vi "calc_jumpTrainWaveform_v0.03.vi"(0 "New input cluster":T1={"Which Position to use for Experiment"=enum."Jumper Safe Position", "Start Position (N)"="", "Jump Position (m)"="", "Duration (s)"=0.0, "Delay (s)"=0.0, "Pulse Width (s)"=0.0, "Valve 1 Position"=0, "Valve 2 Position"=0, "Replicates"=0.0, "Pulse Period (s)"=0.0, "Vholding (mV)"=1.0, "Number of Pulses"=1.0, "valve 1 used now?"=FALSE, "valve 2 used now?"=FALSE, "valve 3 used now? "=FALSE, "Valve 3 Position"=1, "protocol Preview"=[]} {"Valve 3 Position" min=1 max=8; "Number of Pulses" min=1.0 max=8.0; "Vholding (mV)" min=1.0 max=8.0}, 1 "Clear Waveform?":bool, 5 "Old input cluster":T1={"Which Position to use for Experiment"=enum."Jumper Safe Position", "Start Position (N)"="", "Jump Position (m)"="", "Duration (s)"=0.0, "Delay (s)"=0.0, "Pulse Width (s)"=0.0, "Valve 1 Position"=0, "Valve 2 Position"=0, "Replicates"=0.0, "Pulse Period (s)"=0.0, "Vholding (mV)"=1.0, "Number of Pulses"=1.0, "valve 1 used now?"=FALSE, "valve 2 used now?"=FALSE, "valve 3 used now? "=FALSE, "Valve 3 Position"=1, "protocol Preview"=[]} {"Valve 3 Position" min=1 max=8; "Number of Pulses" min=1.0 max=8.0; "Vholding (mV)" min=1.0 max=8.0}, 7 "sample freq":i32=10000, 9 "Jump Filter Freq (Hz)":dbl=30.0, 11 "error in":errorcluster) -> (4 "output cluster":T1={"Which Position to use for Experiment"=enum."Jumper Safe Position", "Start Position (N)"="", "Jump Position (m)"="", "Duration (s)"=0.0, "Delay (s)"=0.0, "Pulse Width (s)"=0.0, "Valve 1 Position"=0, "Valve 2 Position"=0, "Replicates"=0.0, "Pulse Period (s)"=0.0, "Vholding (mV)"=1.0, "Number of Pulses"=1.0, "valve 1 used now?"=FALSE, "valve 2 used now?"=FALSE, "valve 3 used now? "=FALSE, "Valve 3 Position"=1, "protocol Preview"=[]} {"Valve 3 Position" min=1 max=8; "Number of Pulses" min=1.0 max=8.0; "Vholding (mV)" min=1.0 max=8.0}, 15 "error out":errorcluster)   [LabVIEW 2019]
uses:
  <vilib>/Analysis/3filter.llb/Filter Passband Type.ctl
  <vilib>/Analysis/3filter.llb/Bessel Filter (DBL).vi
  <vilib>/measure/NI_MABase.lvlib
  <vilib>/Analysis/NI_AALBase.lvlib
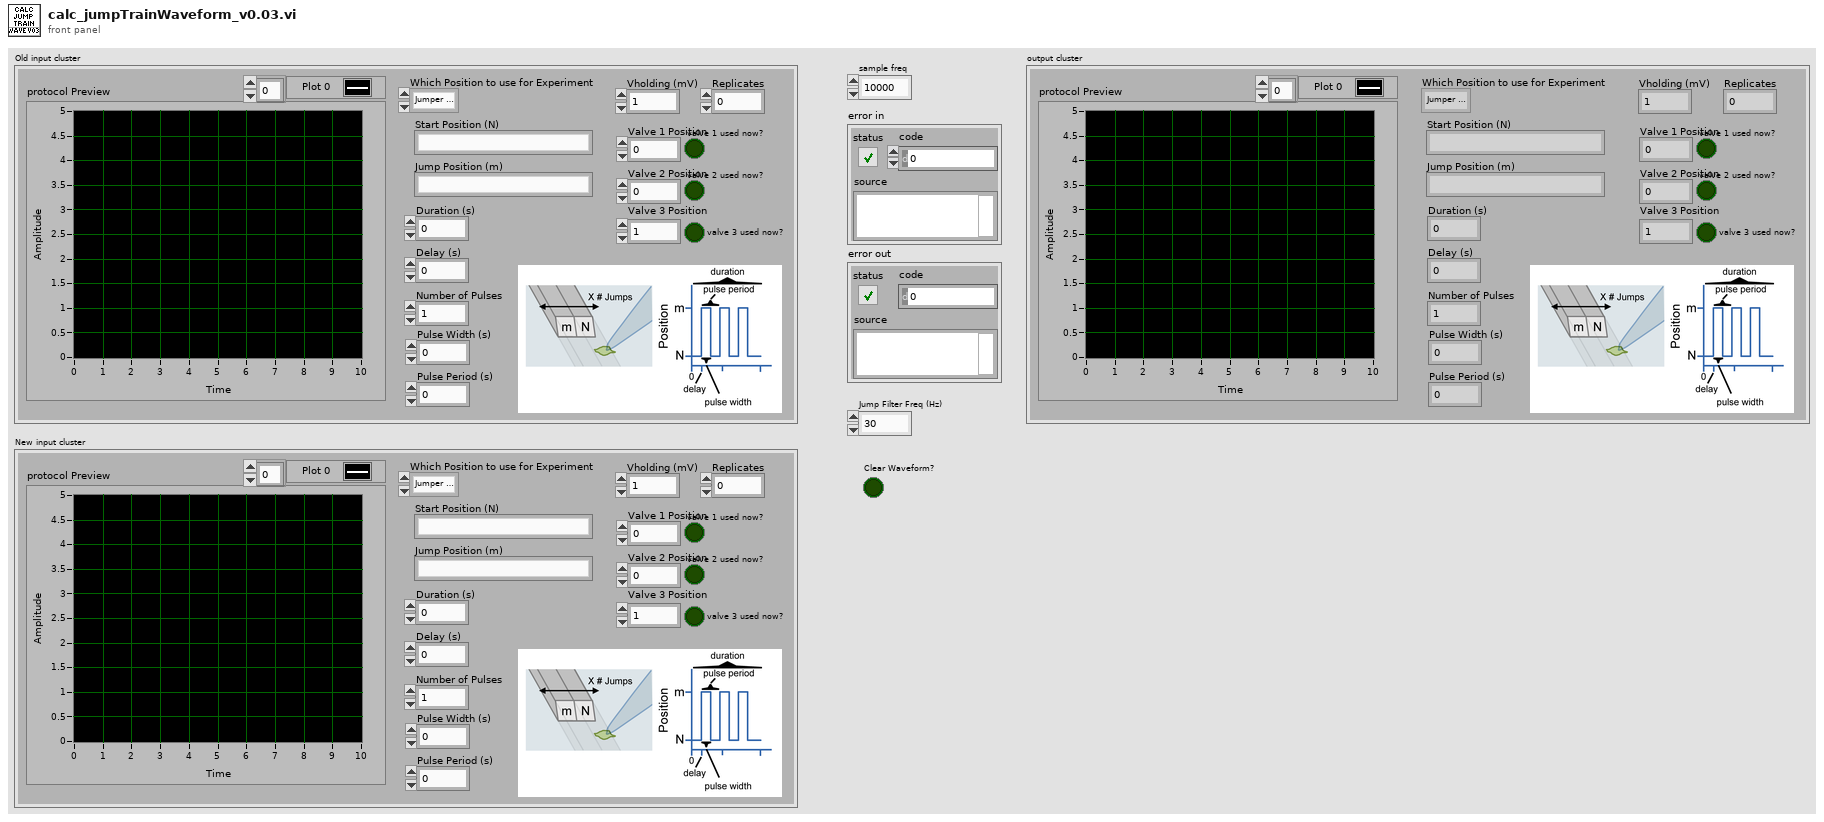
[diagram p1: front panel]
types:
  T1 = cluster{"Which Position to use for Experiment":enum16{"Jumper Safe Position", "Experiment Safe Position", "Jumper Position A", "Jumper Position B", "Jumper Position C", "Jumper Position o-A", "Jumper Position A-o", "Jumper Position A-B", "Jumper Position B-A", "Jumper Position B-C", "Jumper Position C-B", "Jumper Position C-o", "Jumper Position o-C", "Don't Move"}, "Start Position (N)":string, "Jump Position (m)":string, "Duration (s)":dbl, "Delay (s)":dbl, "Pulse Width (s)":dbl, "Valve 1 Position":i16, "Valve 2 Position":i16, "Replicates":dbl, "Pulse Period (s)":dbl, "Vholding (mV)":dbl, "Number of Pulses":dbl, "valve 1 used now?":bool, "valve 2 used now?":bool, "valve 3 used now? ":bool, "Valve 3 Position":i16, "protocol Preview":waveform(dbl)[]}
  T2 = typedef "NI_AALBase.lvlib/Filter Passband Type.ctl" = enum32{"Lowpass", "Highpass", "Bandpass", "Bandstop"}
  T3 = enum16{"Jumper Safe Position", "Experiment Safe Position", "Jumper Position A", "Jumper Position B", "Jumper Position C", "Jumper Position o-A", "Jumper Position A-o", "Jumper Position A-B", "Jumper Position B-A", "Jumper Position B-C", "Jumper Position C-B", "Jumper Position C-o", "Jumper Position o-C", "Don't Move"}
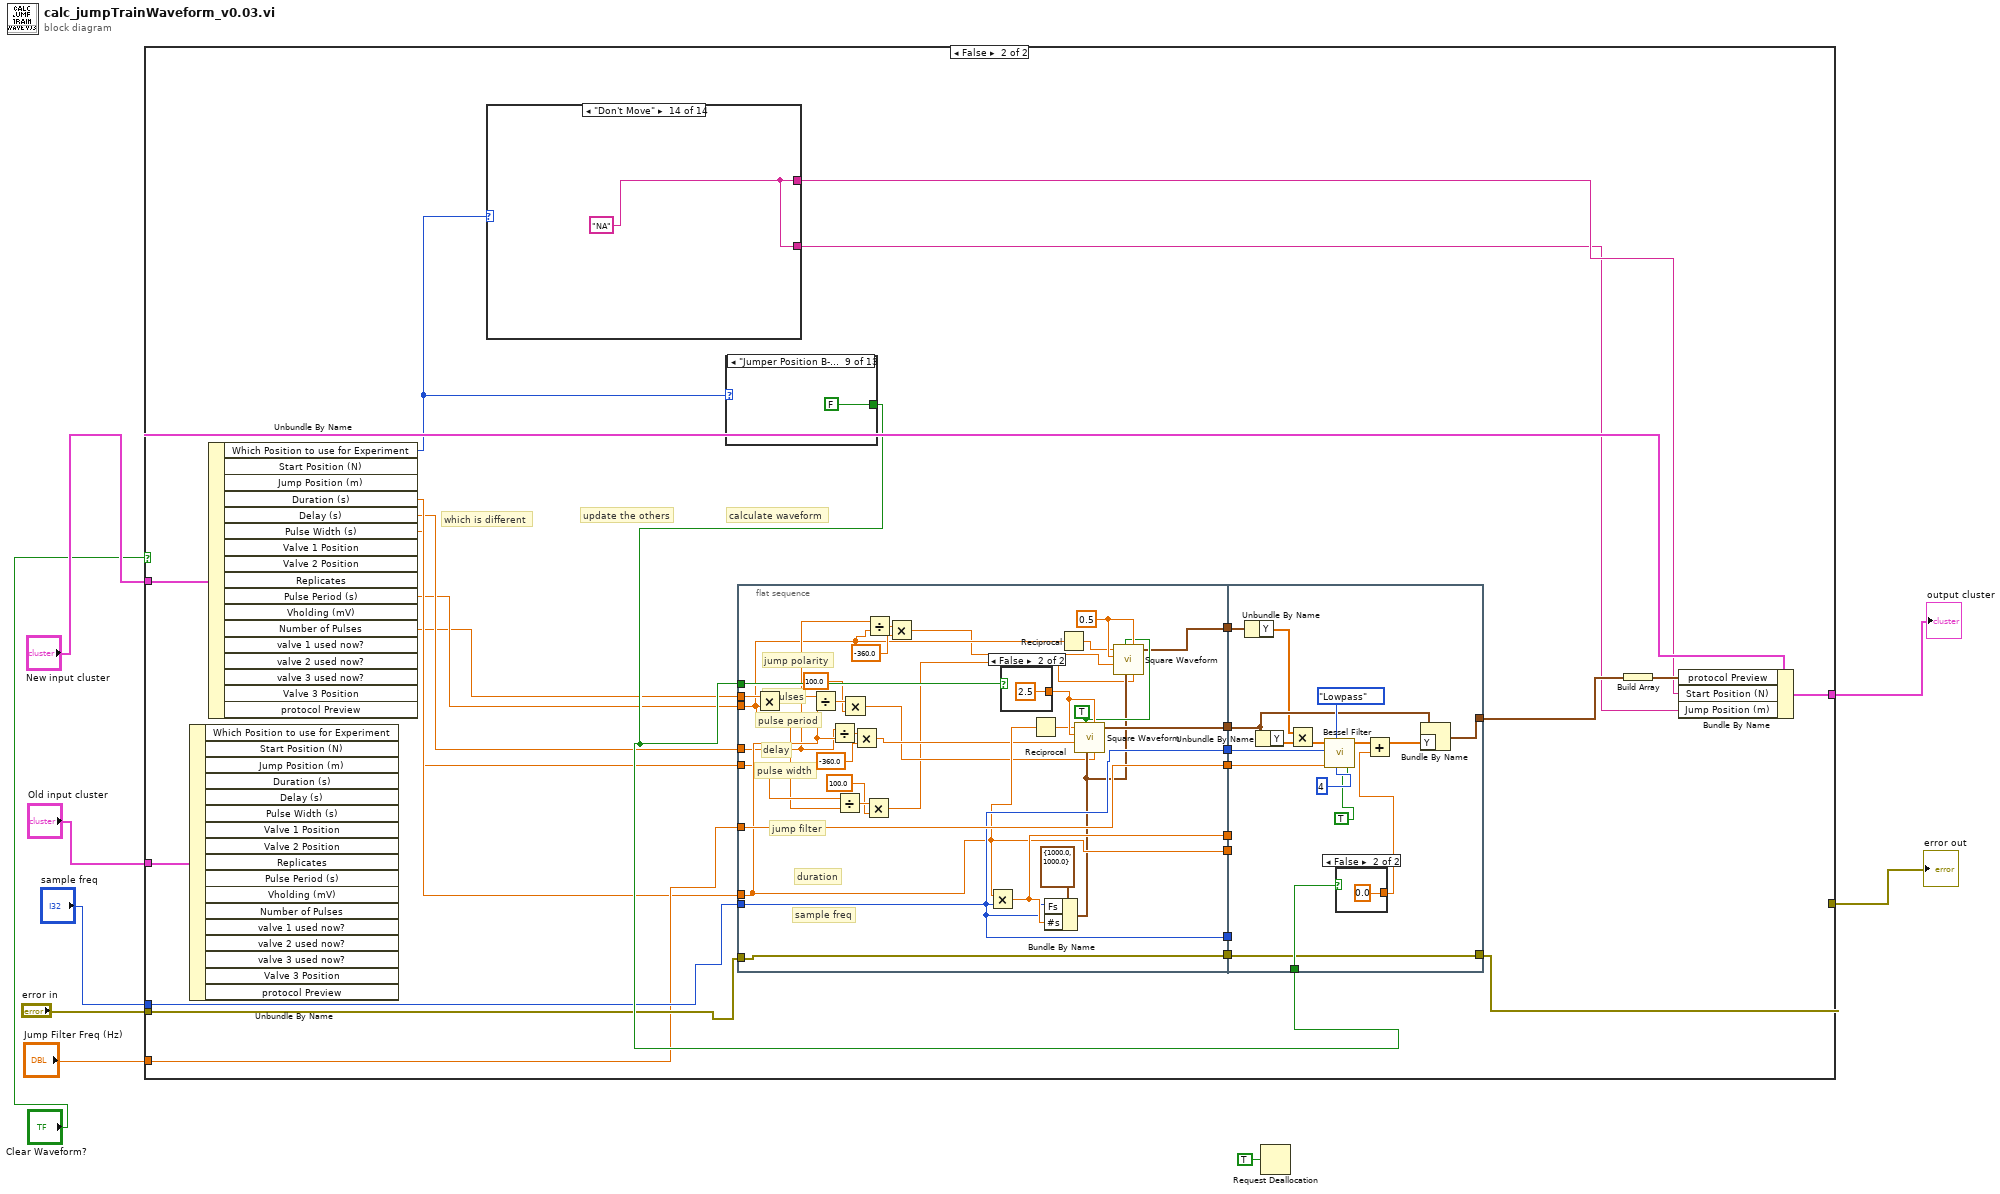
[diagram p0: block diagram]
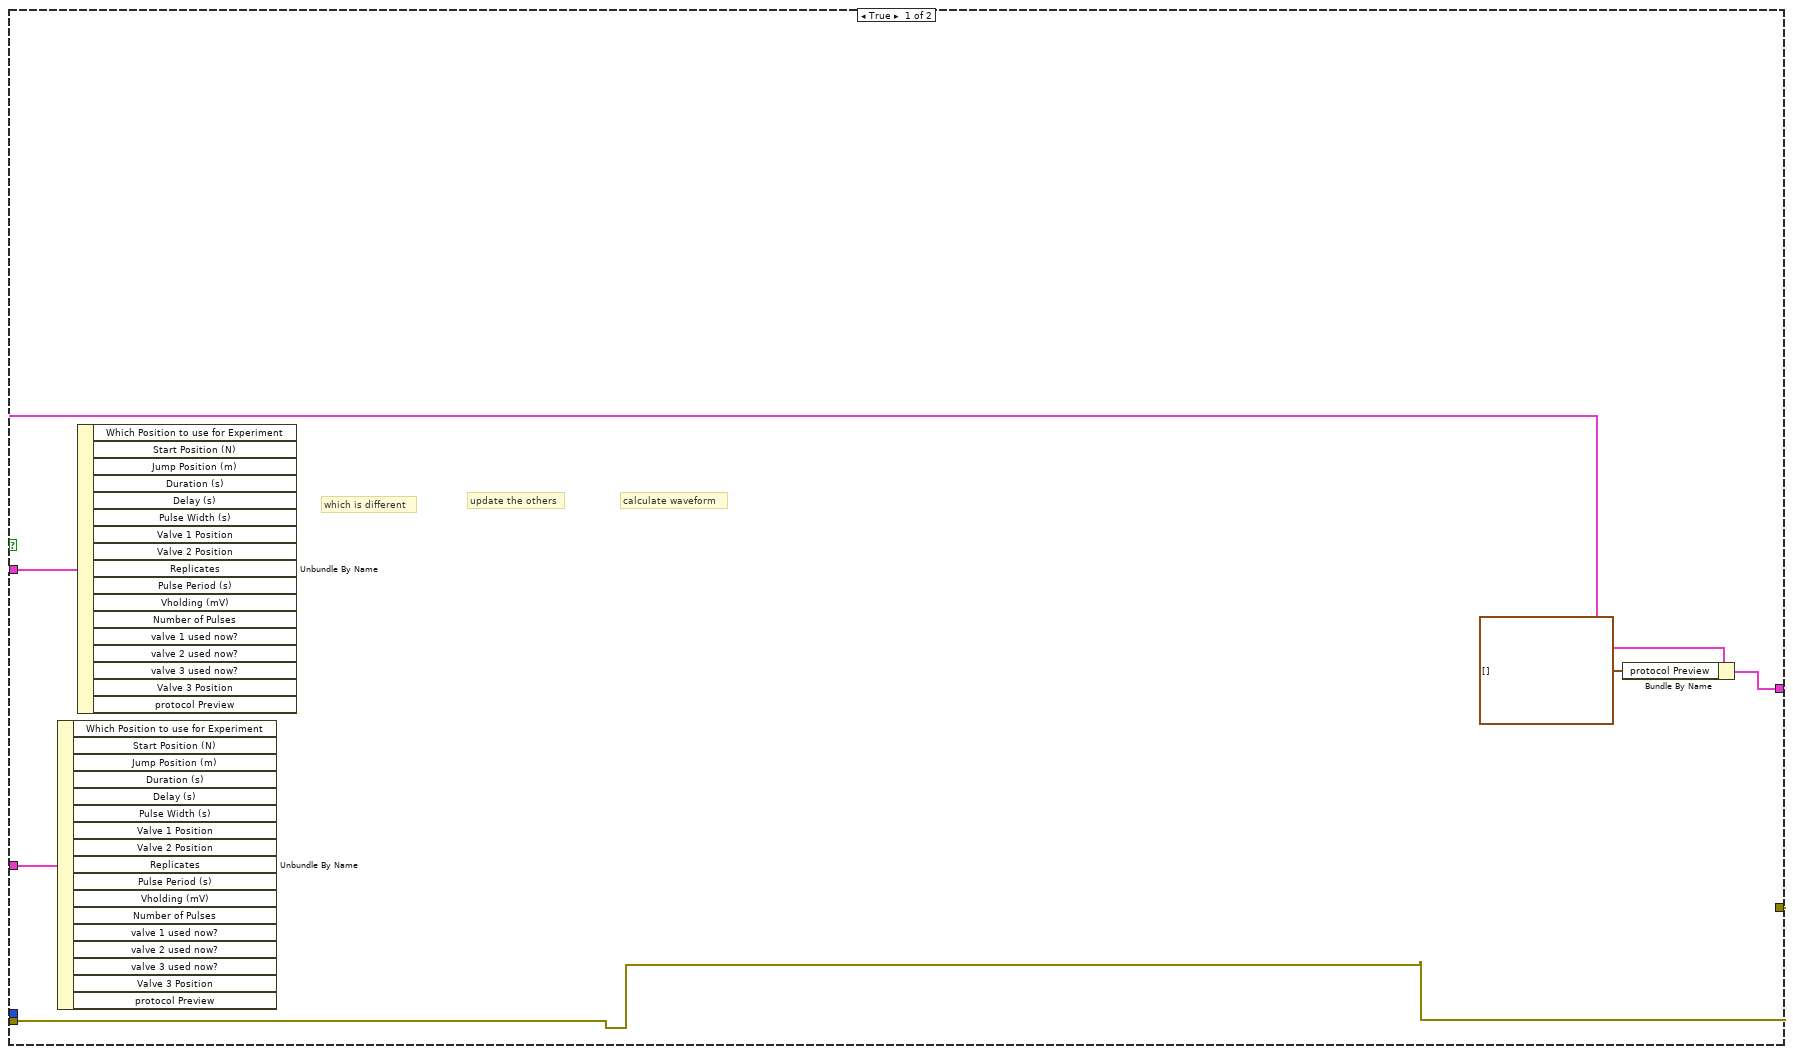
[diagram p2: hidden frame]
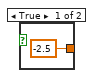
[diagram p3: hidden frame]
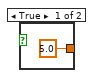
[diagram p4: hidden frame]
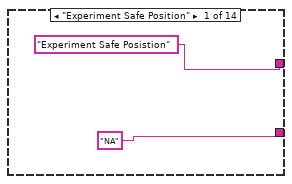
[diagram p5: hidden frame]
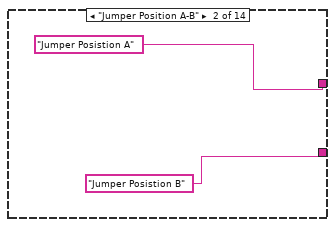
[diagram p6: hidden frame]
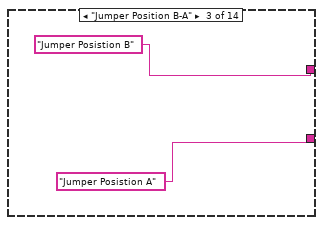
[diagram p7: hidden frame]
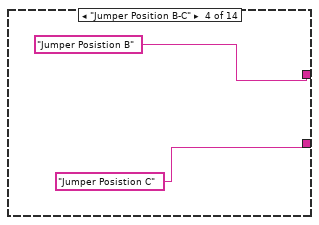
[diagram p8: hidden frame]
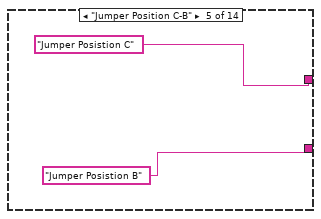
[diagram p9: hidden frame]
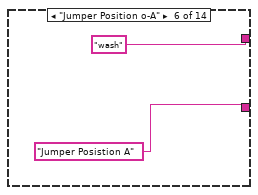
[diagram p10: hidden frame]
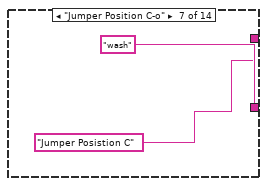
[diagram p11: hidden frame]
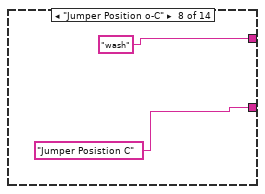
[diagram p12: hidden frame]
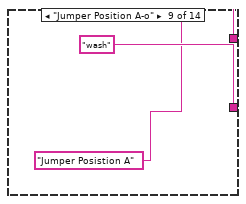
[diagram p13: hidden frame]
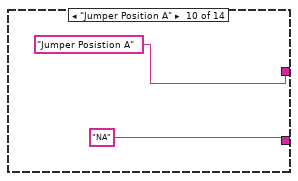
[diagram p14: hidden frame]
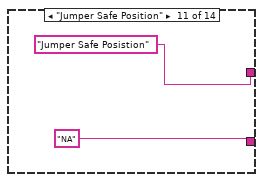
[diagram p15: hidden frame]
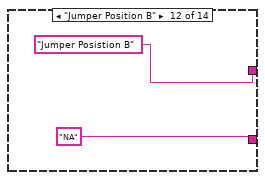
[diagram p16: hidden frame]
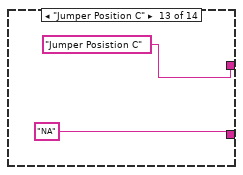
[diagram p17: hidden frame]
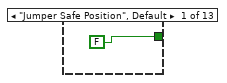
[diagram p18: hidden frame]
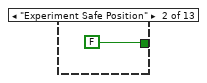
[diagram p19: hidden frame]
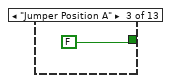
[diagram p20: hidden frame]
diagram:
  n1 = case shown="False" "Clear Waveform?" {
    tunnel: "New input cluster" -> [w14 w32]
    tunnel: [w13 w31] -> w8
    tunnel: "Old input cluster" -> [w12 w30]
    tunnel: "error in" -> [w11 w28]
    tunnel: "sample freq" -> [_ w27]
    tunnel: "Jump Filter Freq (Hz)" -> [_ w26]
    tunnel: [w11 w22] -> w3
    frame True {
      # "calculate waveform"
      # "update the others"
      # "which is different"
      n2 = Unbundle By Name(w12) -> ()  [unwired: 17 out]
      n3 = Unbundle By Name(w14) -> ()  [unwired: 17 out]
      n4 = Bundle By Name(cluster=w14, "protocol Preview"=waveform(dbl)[] []) -> (w13:T1)
    }
    frame False {
      # "calculate waveform"
      # "update the others"
      # "which is different"
      n5 = Unbundle By Name(w30) -> ()  [unwired: 17 out]
      n6 = Unbundle By Name(w32) -> ("Which Position to use for Experiment"=w17:T3, "Duration (s)"=w25:dbl, "Delay (s)"=w24:dbl, "Pulse Width (s)"=w23:dbl, "Pulse Period (s)"=w20:dbl, "Number of Pulses"=w19:dbl)  [unwired: 11 out]
      n7 = case shown="\"Don't Move\"" w17 {
        tunnel: ["Experiment Safe Posistion" "Jumper Posistion A" "Jumper Posistion B" "Jumper Posistion B" "Jumper Posistion C" "wash" "Jumper Posistion C" "wash" "Jumper Posistion A" "Jumper Posistion A" "Jumper Safe Posistion" "Jumper Posistion B" "Jumper Posistion C" w119] -> w16
        tunnel: ["NA" "Jumper Posistion B" "Jumper Posistion A" "Jumper Posistion C" "Jumper Posistion B" "Jumper Posistion A" "wash" "Jumper Posistion C" "wash" "NA" "NA" "NA" "NA" w119] -> w15
        frame "Experiment Safe Position" {
        }
        frame "Jumper Position A-B" {
        }
        frame "Jumper Position B-A" {
        }
        frame "Jumper Position B-C" {
        }
        frame "Jumper Position C-B" {
        }
        frame "Jumper Position o-A" {
        }
        frame "Jumper Position C-o" {
        }
        frame "Jumper Position o-C" {
        }
        frame "Jumper Position A-o" {
        }
        frame "Jumper Position A" {
        }
        frame "Jumper Safe Position" {
        }
        frame "Jumper Position B" {
        }
        frame "Jumper Position C" {
        }
        frame "Don't Move" {
          w119 = "NA"
        }
      }
      n8 = case shown="\"Jumper Position B-A\"" w17 {
        tunnel: [FALSE FALSE FALSE FALSE FALSE TRUE FALSE TRUE FALSE TRUE FALSE TRUE FALSE] -> w29
        frame "Jumper Safe Position", Default {
        }
        frame "Experiment Safe Position" {
        }
        frame "Jumper Position A" {
        }
        frame "Jumper Position B" {
        }
        frame "Jumper Position C" {
        }
        frame "Jumper Position o-A" {
        }
        frame "Jumper Position A-o" {
        }
        frame "Jumper Position A-B" {
        }
        frame "Jumper Position B-A" {
        }
        frame "Jumper Position B-C" {
        }
        frame "Jumper Position C-B" {
        }
        frame "Jumper Position C-o" {
        }
        frame "Jumper Position o-C" {
        }
      }
      n9 = flat-sequence {
        tunnel: w25 -> [w60]
        tunnel: w26 -> [w70]
        tunnel: w27 -> [w69]
        tunnel: [w71] -> w40
        tunnel: [w69] -> w39
        tunnel: [w70] -> w38
        tunnel: [w69] -> w37
        tunnel: [w68] -> w36
        tunnel: w28 -> [w67]
        tunnel: [w67] -> w35
        tunnel: w29 -> [w66]
        tunnel: [w60] -> w34
        tunnel: w19 -> [w58]
        tunnel: w20 -> [w42]
        tunnel: w24 -> [w43]
        tunnel: w23 -> [w51]
        tunnel: [w50] -> w33
        tunnel: w40 -> [_]
        tunnel: w39 -> [_]
        tunnel: w38 -> [w87]
        tunnel: w37 -> [w86]
        tunnel: w36 -> [w85]
        tunnel: w35 -> [w77]
        tunnel: w29 -> [w82]
        tunnel: w34 -> [_]
        tunnel: w33 -> [w80]
        tunnel: [w77] -> w22
        tunnel: [w76] -> w21
        frame #0 {
          w56 = 0.5 ("Amplitude")
          w55 = TRUE ("reset signal")
          # "sample freq"
          # "duration"
          # "jump filter"
          # "pulse width"
          # "delay"
          # "pulse period"
          # "#pulses"
          # "jump polarity"
          n10 = Multiply(x=w58, y=w42) -> (x*y=w59:dbl)
          n11 = Divide(x=w59, y=w60) -> (x/y=w64:dbl)
          n12 = Divide(x=w43, y=w60) -> (x/y=w61:dbl)
          n13 = Divide(x=w51, y=w42) -> (x/y=w53:dbl)
          n14 = Multiply(x=w64, y=100.0) -> (x*y=w47:dbl)
          n15 = Multiply(x=w61, y=-360.0) -> (x*y=w54:dbl)
          n16 = Multiply(x=w53, y=100.0) -> (x*y=w46:dbl)
          n17 = Divide(x=w43, y=w42) -> (x/y=w45:dbl)
          n18 = Multiply(x=w45, y=-360.0) -> (x*y=w41:dbl)
          n19 = Multiply(x=w60, y=w69) -> (x*y=w71:dbl)
          n20 = case shown="False" w66 {
            tunnel: [-2.5 ("Amplitude") 2.5 ("Amplitude")] -> w65
            frame True {
            }
            frame False {
            }
          }
          n21 = Reciprocal(x=w60) -> (1/x=w57:dbl)
          n22 = Bundle By Name(cluster=cluster{"Fs":dbl, "#s":dbl} {"Fs"=1000.0, "#s"=1000.0} ("sampling info"), "Fs"=w69, "#s"=w71) -> (w49:cluster{"Fs":dbl, "#s":dbl})
          n23 = Reciprocal(x=w42) -> (1/x=w48:dbl)
          n24 = call <vilib>:"Square Waveform.vi"("duty cycle (%)"=w47, "offset"=w65, "sampling info"=w49, "reset signal"=w55, "phase"=w54, "amplitude"=w65, "frequency"=w57) -> ("signal out"=w68:waveform(dbl))  [unwired: 3 in, 1 out]
          n25 = call <vilib>:"Square Waveform.vi"("duty cycle (%)"=w46, "offset"=w56, "sampling info"=w49, "reset signal"=w55, "phase"=w41, "amplitude"=w56, "frequency"=w48) -> ("signal out"=w50:waveform(dbl))  [unwired: 3 in, 1 out]
        }
        frame #1 {
          n26 = Unbundle By Name(w80) -> ("Y"=w78:dbl[])
          n27 = Unbundle By Name(w85) -> ("Y"=w90:dbl[])
          n28 = Multiply(x=w78, y=w90) -> (x*y=w79:dbl[])
          n29 = call-poly <vilib>:"Bessel Filter.vi"("init/cont (init:F)"=TRUE, "order"=4, "filter type"=Filter_Passband_Type."Lowpass", "low cutoff freq: fl"=w87, "sampling freq: fs"=w86, "X"=w79) -> ("Filtered X"=w88:dbl[])  [unwired: 2 in, 1 out]
          n30 = case shown="False" w82 {
            tunnel: [5.0 ("Amplitude") 0.0 ("Amplitude")] -> w81
            frame True {
            }
            frame False {
            }
          }
          n31 = Add(x=w88, y=w81) -> (x+y=w83:dbl[])
          n32 = Bundle By Name(cluster=w85, "Y"=w83) -> (w76:waveform(dbl))
        }
      }
      n33 = Build Array(w21) -> (w18:waveform(dbl)[])
      n34 = Bundle By Name(cluster=w32, "protocol Preview"=w18, "Start Position (N)"=w16, "Jump Position (m)"=w15) -> (w31:T1)
    }
  }
  "output cluster" <- w8
  "error out" <- w3
  n35 = Request Deallocation(TRUE ("flag")) -> ()
